vi "Prior.vi"(0 "reference in":refnum<class "CustomersBase.lvclass">, 5 "error in (no error)":errorcluster) -> (14 "reference out":refnum<class "CustomersBase.lvclass">, 19 "error out":errorcluster)   [LabVIEW 2020, in "CustomersBase.lvclass"]
uses:
  CustomersBase.lvclass
  DataObject_class/DataObject.lvclass
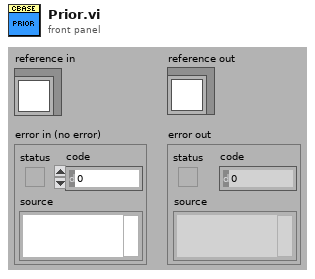
[diagram p1: front panel]
types:
  T1 = typedef "CustomersBase.lvclass/ObjectAttributes.ctl" = cluster{"_dataObject":refnum<class "DataObject.lvclass">, "Group":string}
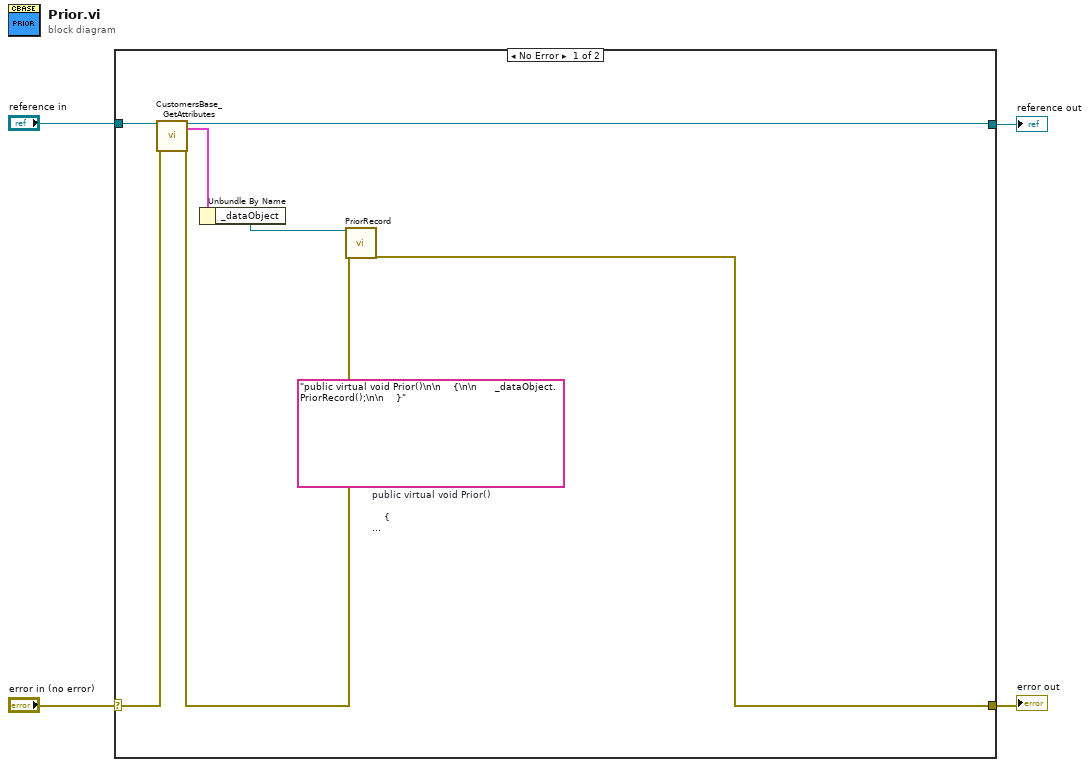
[diagram p0: block diagram]
diagram:
  n1 = case shown="No Error" "error in (no error)" {
    selector: "error in (no error)" -> [w10 w13]
    tunnel: [w5 w13] -> w3
    tunnel: [w8 w12] -> w1
    tunnel: "reference in" -> [w11 w12]
    frame No Error {
      (unwired) "public virtual void Prior()\n\n    {\n\n      _dataObject.PriorRecord();\n\n    }"  # public virtual void Prior()      {        _dataObject.PriorRecord();      }
      n2 = call "CustomersBase_GetAttributes.vi"("reference in"=w11, "error in (no error)"=w10) -> ("reference out"=w8:refnum<class "CustomersBase.lvclass">, "Data"=w9:T1, "error out"=w6:errorcluster)  [unwired: 14 in, 1 out]
      n3 = Unbundle By Name(w9) -> ("_dataObject"=w7:refnum<class "DataObject.lvclass">)
      n4 = call-dynamic "PriorRecord.vi"("reference in"=w7, "error in (no error)"=w6) -> ("error out"=w5:errorcluster)  [unwired: 16 in, 1 out]
    }
    frame Error {
    }
  }
  "error out" <- w3
  "reference out" <- w1
